vi "TiposdeDatos.vi"() -> ()   [LabVIEW 2020]
panel:
  in  "LabVIEW Object 2":refnum<class>
  out "LabVIEW Object":refnum<class>
  in  "Variant 2":variant
  out "Variant":variant
  in  "Cluster 2":T1 {"Meter" scale=0.0..10.0; "Thermometer" scale=0.0..100.0}
  out "Cluster":T1 {"Meter" scale=0.0..10.0; "Thermometer" scale=0.0..100.0}
  in  "Array 4":string[](array[string])
  in  "Array 3":bool[](array[boolean])
  in  "Array 2":u16[](array[slide]) scale=0.0..100.0
  in  "Array":dbl[](array[slide]) scale=0.0..10.0
  out "String 2":string
  in  "String":string
  out "Boolean 2":bool
  in  "Boolean":bool
  out "Tank":u8(slide) scale=0.0..10.0
  in  "Dial":u8(knob) scale=0.0..10.0
  out "Thermometer":dbl(slide) scale=0.0..10.0
  in  "Knob":dbl(knob) scale=0.0..10.0
  # "Tipos de Datos"
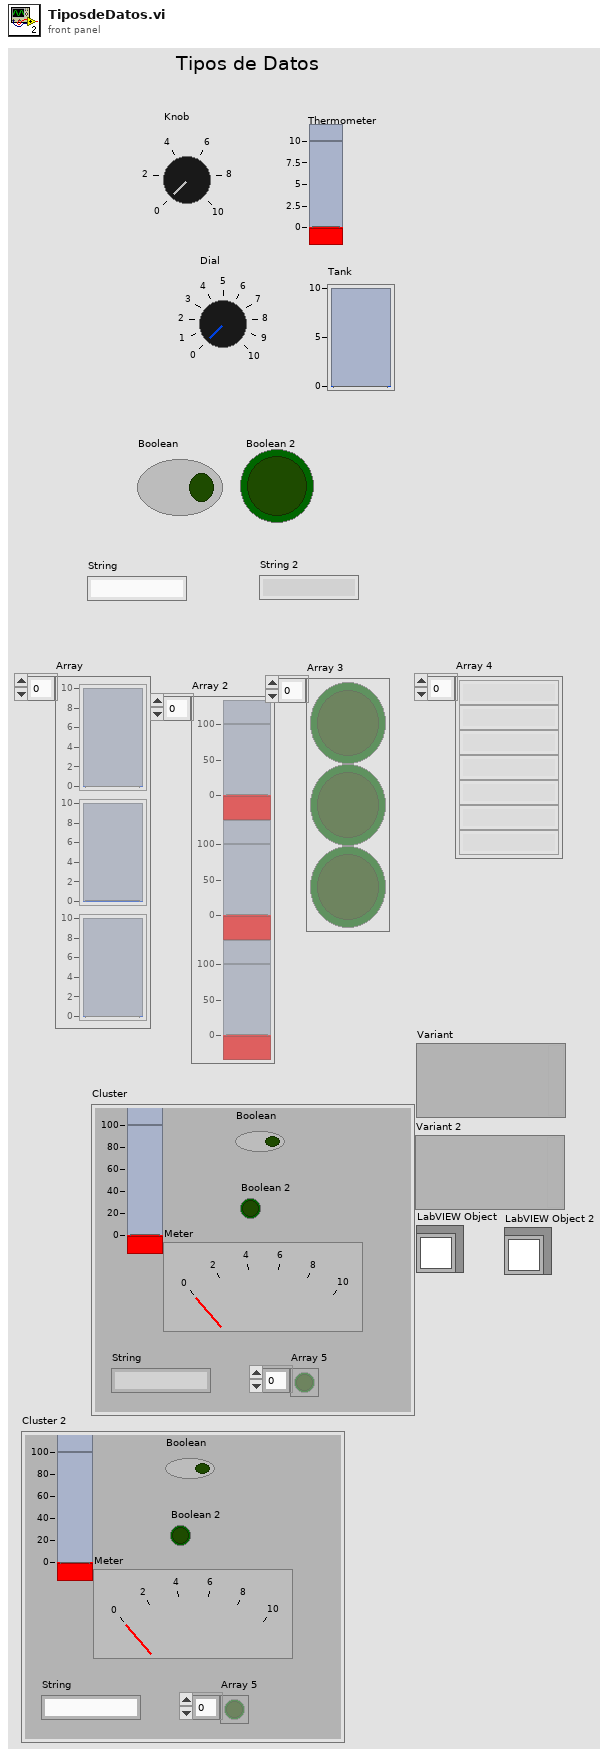
[diagram p1: front panel]
types:
  T1 = cluster{"Thermometer":dbl, "Boolean":bool, "Boolean 2":bool, "Meter":dbl, "String":string, "Array 5":bool[]}
  T2 = cluster{cluster{string, dbl[]}, cluster{string[], bool[], i32}}
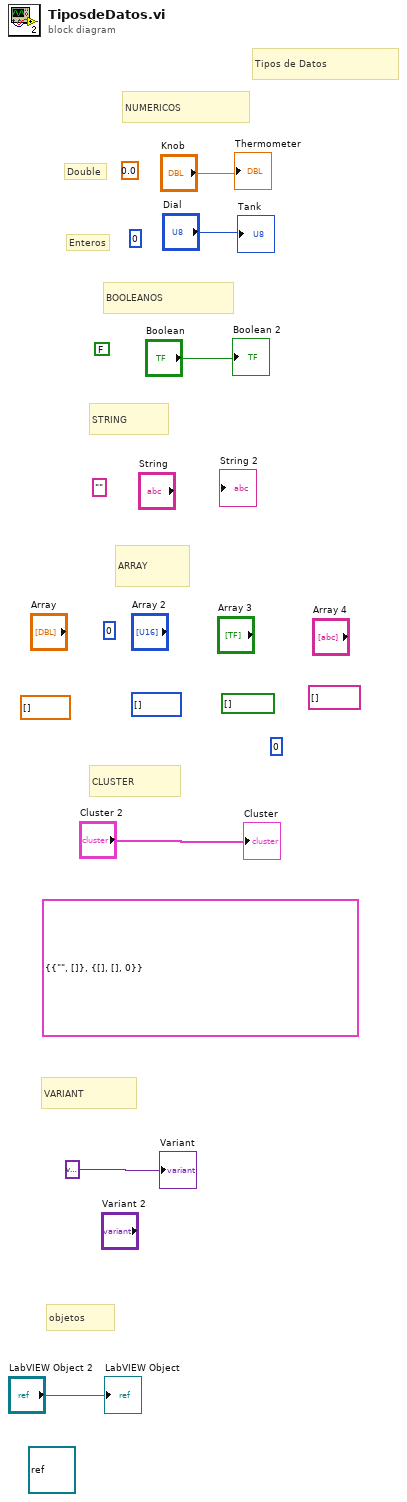
[diagram p0: block diagram]
diagram:
  (unwired) refnum<class> refnum ("LabVIEW Object 2")
  (unwired) 0
  (unwired) T2 {{"", []}, {[], [], 0}}
  (unwired) 0
  (unwired) string[] []
  (unwired) bool[] []
  (unwired) i32[] []
  (unwired) dbl[] []
  (unwired) ""
  (unwired) FALSE
  (unwired) 0
  (unwired) 0.0
  # "objetos"
  # "Enteros"
  # "Double"
  # "VARIANT"
  # "CLUSTER"
  # "ARRAY"
  # "STRING"
  # "BOOLEANOS"
  # "NUMERICOS"
  # "Tipos de Datos"
  "Thermometer" <- "Knob"
  "Tank" <- "Dial"
  "Boolean 2" <- "Boolean"
  "Cluster" <- "Cluster 2"
  "Variant" <- variant
  "LabVIEW Object" <- "LabVIEW Object 2"
